vi "ReversedEngineering GetCaseStringConstants.vi"(0 "Diagram":refnum<vi>, 5 "error in (no error)":errorcluster) -> (15 "StringConstants":string[](array[string]), 16 "EventStructureUsed":bool, 19 "error out":errorcluster)   [LabVIEW 2012]
uses:
  <resource>/Framework/Providers/Open_GDS/UML/ReversedEngineering/ReversedEngineering QueuedStateMachinMemoryAction.ctl
panel:
  in  "Debug?":bool
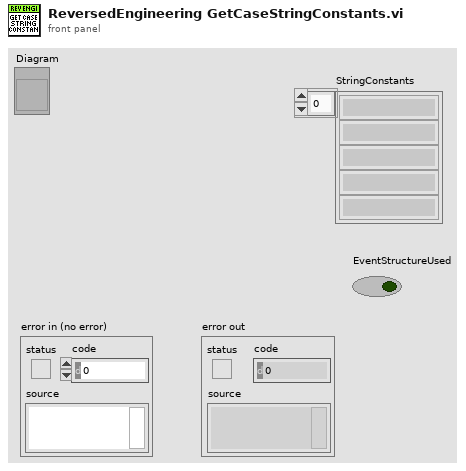
[diagram p1: front panel]
types:
  T1 = typedef "ReversedEngineering QueuedStateMachinMemoryAction.ctl" = enum16{"Initialize", "GetInsertQueuedArrayElementsVI", "SetQueuedStateJumps", "GetQueuedStateJumps"}
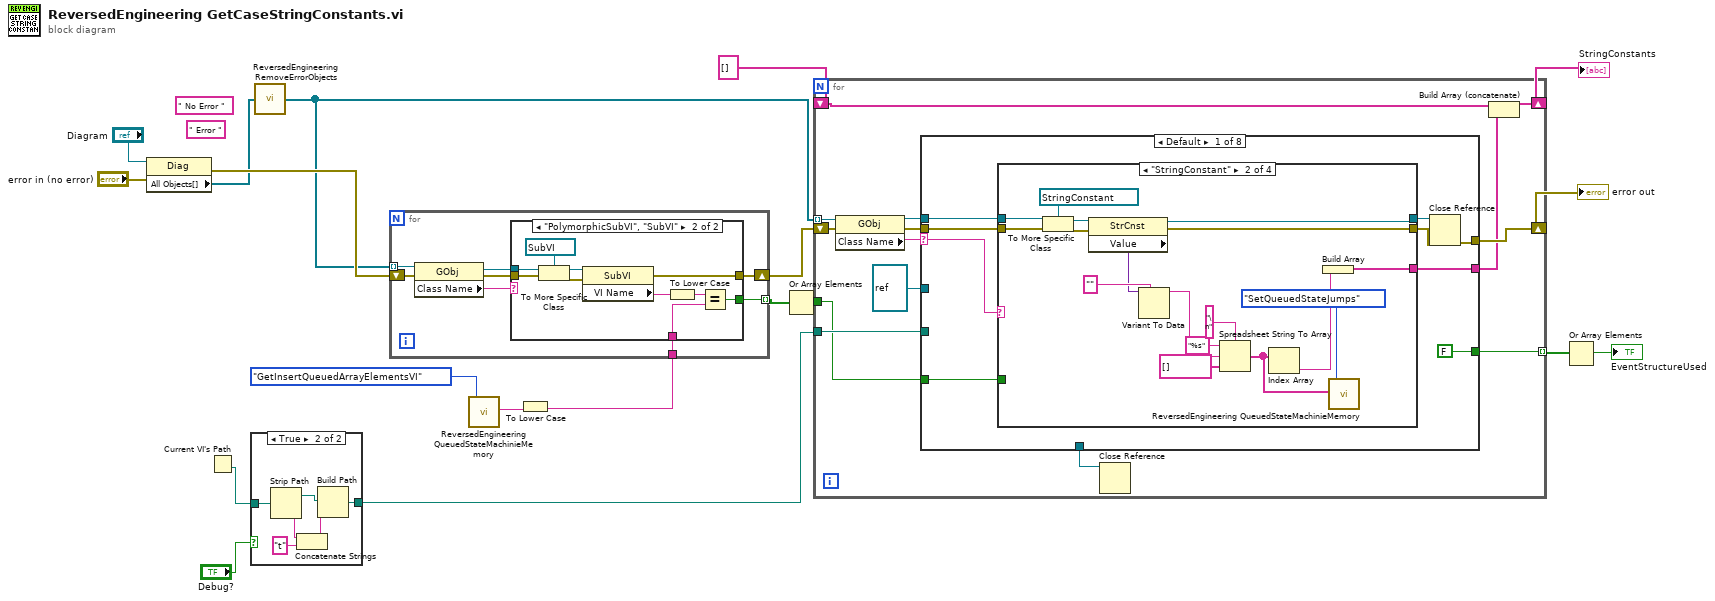
[diagram p0: block diagram]
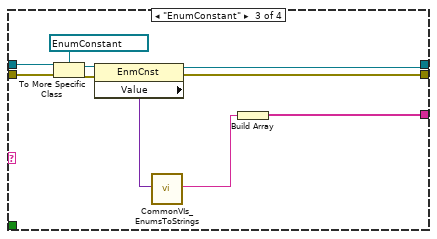
[diagram p5: hidden frame]
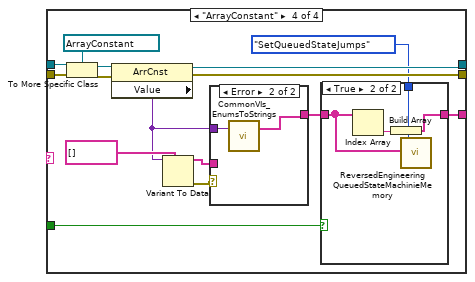
[diagram p6: hidden frame]
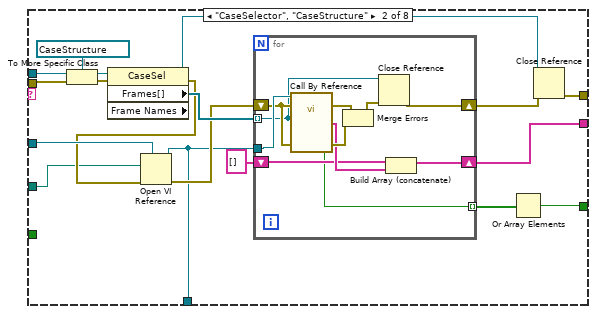
[diagram p9: hidden frame]
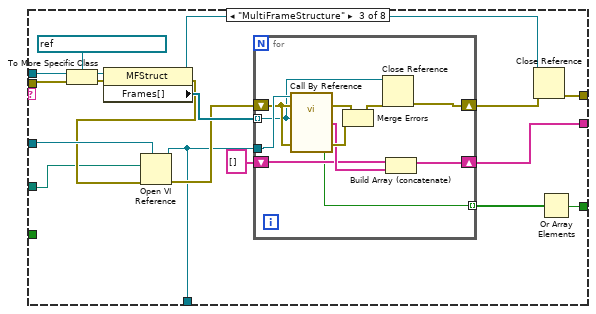
[diagram p10: hidden frame]
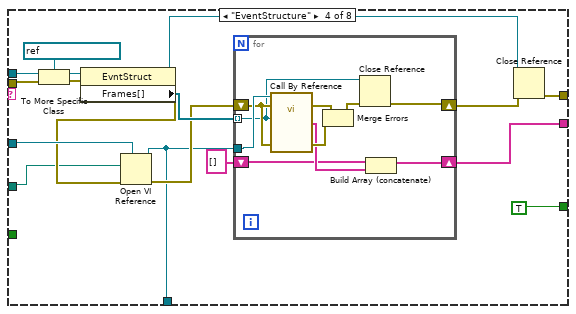
[diagram p11: hidden frame]
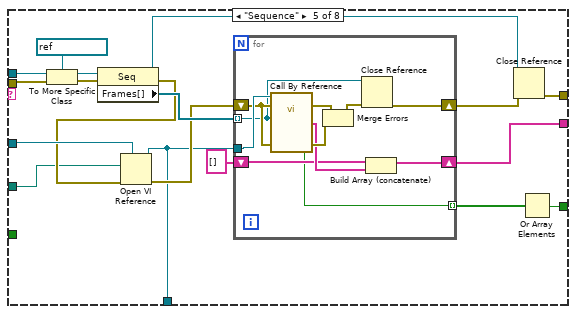
[diagram p12: hidden frame]
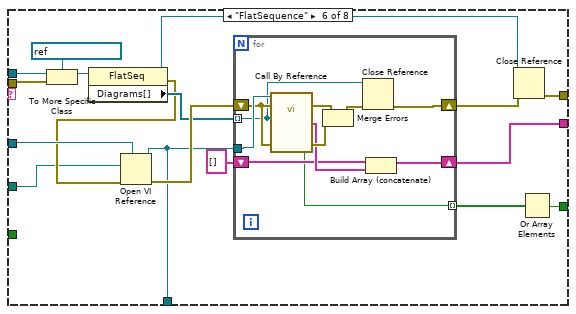
[diagram p13: hidden frame]
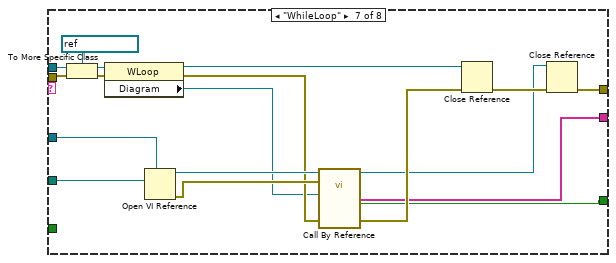
[diagram p14: hidden frame]
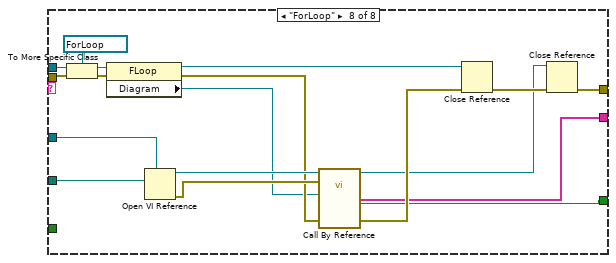
[diagram p15: hidden frame]
diagram:
  (unwired) " Error "
  (unwired) " No Error "
  n1 = property class="Diag"(reference="Diagram", error in="error in (no error)") -> (error out=w6:errorcluster, "All Objects[]"=w2:refnum<vi>[])  [unwired: 1 out]
  n2 = Current VI's Path() -> (path=w14:path)
  n3 = case shown="True" "Debug?" {
    tunnel: w14 -> [w20 w25]
    tunnel: [w20 w24] -> w13
    frame False {
    }
    frame True {
      n4 = Strip Path(path=w25) -> (stripped path=w26:path, name=w23:string)
      n5 = Concatenate Strings(w23, "t" ("string")) -> (w22:string)
      n6 = Build Path(base path=w26, name or relative path=w22) -> (appended path=w24:path)
    }
  }
  n7 = call <resource>:"ReversedEngineering RemoveErrorObjects.vi"("ObjectsIn"=w2) -> ("ObjectsOut"=w1:refnum<vi>[])
  n8 = call <resource>:"ReversedEngineering QueuedStateMachinieMemory.vi"("Action(GetInsertQueuedArrayElementsVI)"=ReversedEngineering_QueuedStateMachinMemoryAction."GetInsertQueuedArrayElementsVI" ("Action(GetInsertQueuedArrayElements)")) -> ("VIName"=w8:string)  [unwired: 3 in, 15 out]
  n9 = To Lower Case(string=w8) -> (all lower case string=w7:string)
  n10 = for {
    tunnel: w1 -> [w34] mode=indexing
    shift-right: [w27] -> w5
    shift-left: w6 -> [w32]
    tunnel: w7 -> [w29]
    tunnel: [w28] -> w4 mode=indexing
    n11 = property class="GObj"(reference=w34, error in=w32) -> (reference out=w31:refnum<vi>, error out=w30:errorcluster, "Class Name"=w33:string)
    n12 = case shown="\"PolymorphicSubVI\", \"SubVI\"" w33 {
      tunnel: w31 -> [_ w45]
      tunnel: w30 -> [w35 w43]
      tunnel: w29 -> [_ w39]
      tunnel: [_ w38] -> w28
      tunnel: [w35 w37] -> w27
      frame "False", Default {
      }
      frame "PolymorphicSubVI", "SubVI" {
        n13 = To More Specific Class(target class=refnum<vi> refnum ("WhileLoop"), reference=w45, error in=w43) -> (specific class reference=w42:refnum<vi>, error out=w36:errorcluster)
        n14 = property class="SubVI"(reference=w42, error in=w36) -> (error out=w37:errorcluster, "VI Name"=w41:string)  [unwired: 1 out]
        n15 = To Lower Case(string=w41) -> (all lower case string=w40:string)
        n16 = Equal?(x=w40, y=w39) -> (x = y?=w38:bool)
      }
    }
  }
  n17 = Or Array Elements(Boolean array=w4) -> (logical OR=w3:bool)
  n18 = for {
    tunnel: w1 -> [w59] mode=indexing
    shift-right: [w54] -> w17
    shift-left: w5 -> [w56]
    shift-right: [w52] -> w16
    shift-left: string[] [] -> [w53]
    tunnel: w13 -> [w49]
    tunnel: [w47] -> w11 mode=indexing
    tunnel: w3 -> [w46]
    n19 = property class="GObj"(reference=w59, error in=w56) -> (reference out=w57:refnum<vi>, error out=w55:errorcluster, "Class Name"=w58:string)
    n20 = case shown="Default" w58 {
      selector: w58 -> [w67 _ _ _ _ _ _ _]
      tunnel: w57 -> [w65 w138 w167 w195 w223 w251 w280 w298]
      tunnel: w55 -> [w66 w133 w163 w192 w219 w250 w274 w292]
      tunnel: [w68 w132 w162 w191 w218 w249 w266 w284] -> w54
      tunnel: [w62 w126 w156 w185 w213 w245 w269 w287] -> w51
      tunnel: refnum<vi> refnum ("VI Refnum") -> [_ w129 w159 w188 w215 w247 w268 w286]
      tunnel: w49 -> [_ w124 w153 w182 w210 w238 w264 w282]
      tunnel: [_ w123 w152 w181 w208 w237 _ _] -> w48
      tunnel: [FALSE ("EventStructureUsed") w121 w151 TRUE w207 w236 w263 w281] -> w47
      tunnel: w46 -> [w60 _ _ _ _ _ _ _]
      frame Default {
        n21 = case shown="\"StringConstant\"" w67 {
          tunnel: w66 -> [w70 w85 w95 w110]
          tunnel: w65 -> [w69 w86 w96 w111]
          tunnel: [w70 w82 w92 w108] -> w64
          tunnel: [w69 w81 w91 w107] -> w63
          tunnel: [_ w83 w93 w99] -> w62
          tunnel: w60 -> [_ _ _ w101]
          frame "False", Default {
          }
          frame "StringConstant" {
            n22 = To More Specific Class(target class=refnum<vi> refnum ("WhileLoop"), reference=w86, error in=w85) -> (specific class reference=w84:refnum<vi>, error out=w80:errorcluster)
            n23 = property class="StrCnst"(reference=w84, error in=w80) -> (reference out=w81:refnum<vi>, error out=w82:errorcluster, "Value"=w78:variant)
            n24 = Variant To Data(type="", Variant=w78) -> (data=w74:string)  [unwired: 1 in, 1 out]
            n25 = Spreadsheet String To Array(delimiter (Tab)="\n", format string="%s", spreadsheet string=w74, array type (2D Dbl)=string[] []) -> (array=w72:string[])
            n26 = Index Array(array=w72) -> (element=w73:string)  [unwired: 1 in]
            n27 = Build Array(w73) -> (w83:string[])
            n28 = call <resource>:"ReversedEngineering QueuedStateMachinieMemory.vi"("StateJumps"=w72, "Action(GetInsertQueuedArrayElementsVI)"=ReversedEngineering_QueuedStateMachinMemoryAction."SetQueuedStateJumps") -> ()  [unwired: 2 in, 16 out]
          }
          frame "EnumConstant" {
            n29 = To More Specific Class(target class=refnum<vi> refnum ("WhileLoop"), reference=w96, error in=w95) -> (specific class reference=w94:refnum<vi>, error out=w90:errorcluster)
            n30 = property class="EnmCnst"(reference=w94, error in=w90) -> (reference out=w91:refnum<vi>, error out=w92:errorcluster, "Value"=w89:variant)
            n31 = call <resource>:"CommonVIs_EnumsToStrings.vi"("SingleEnumVariantIn"=w89) -> ("EnumItem"=w88:string)  [unwired: 2 in, 16 out]
            n32 = Build Array(w88) -> (w93:string[])
          }
          frame "ArrayConstant" {
            n33 = To More Specific Class(target class=refnum<vi> refnum ("WhileLoop"), reference=w111, error in=w110) -> (specific class reference=w109:refnum<vi>, error out=w106:errorcluster)
            n34 = property class="ArrCnst"(reference=w109, error in=w106) -> (reference out=w107:refnum<vi>, error out=w108:errorcluster, "Value"=w103:variant)
            n35 = Variant To Data(type=string[] [], Variant=w103) -> (data=w102:string[], error out=w104:errorcluster)  [unwired: 1 in]
            n36 = case shown="Error" w104 {
              tunnel: w103 -> [_ w120]
              tunnel: w102 -> [w118 _]
              tunnel: [w118 w119] -> w100
              frame No Error {
              }
              frame Error {
                n37 = call <resource>:"CommonVIs_EnumsToStrings.vi"("ArrayEnumVariantIn"=w120) -> ("EnumItems(string)"=w119:string[])  [unwired: 2 in, 16 out]
              }
            }
            n38 = case shown="True" w101 {
              tunnel: w100 -> [w113 w115]
              tunnel: [w113 w116] -> w99
              tunnel: ReversedEngineering_QueuedStateMachinMemoryAction."SetQueuedStateJumps" ("Action(GetInsertQueuedArrayElementsVI)") -> [_ w117]
              frame False {
              }
              frame True {
                n39 = Index Array(array=w115) -> (element=w114:string)  [unwired: 1 in]
                n40 = Build Array(w114) -> (w116:string[])
                n41 = call <resource>:"ReversedEngineering QueuedStateMachinieMemory.vi"("StateJumps"=w115, "Action(GetInsertQueuedArrayElementsVI)"=w117) -> ()  [unwired: 2 in, 16 out]
              }
            }
          }
        }
        n42 = Close Reference(reference=w63, error in (no error)=w64) -> (error out=w68:errorcluster)
      }
      frame "CaseSelector", "CaseStructure" {
        n43 = To More Specific Class(target class=refnum<vi> refnum ("CaseSelector"), reference=w138, error in=w133) -> (specific class reference=w136:refnum<vi>, error out=w134:errorcluster)
        n44 = property class="CaseSel" props=["Frames[]", "Frame Names"](reference=w136, error in=w134) -> (reference out=w130:refnum<vi>, error out=w128:errorcluster, "Frames[]"=w135:refnum<vi>[])  [unwired: 1 out]
        n45 = Open VI Reference(type specifier VI Refnum (for type only)=w129, vi path=w124, error in (no error)=w128) -> (vi reference=w123:refnum<vi>, error out=w131:errorcluster)  [unwired: 3 out]
        n46 = for {
          tunnel: w135 -> [w140] mode=indexing
          shift-right: [w142] -> w127
          shift-left: w131 -> [w147]
          tunnel: w123 -> [w148]
          shift-right: [w143] -> w126
          shift-left: string[] [] -> [w144]
          tunnel: [w139] -> w122 mode=indexing
          n47 = call-by-ref "?"(reference=w148, error in=w147, "Diagram"=w140, "error in (no error)"=w147) -> (error out=w149:errorcluster, "StringConstants"=w145:string[], "EventStructureUsed"=w139:bool, 19:"error out"=w146:errorcluster)  [unwired: 15 in, 1 out]
          n48 = Merge Errors(w149, w146) -> (w141:errorcluster)
          n49 = Close Reference(reference=w140, error in (no error)=w141) -> (error out=w142:errorcluster)
          n50 = Build Array (concatenate)(w144, w145) -> (w143:string[])
        }
        n51 = Or Array Elements(Boolean array=w122) -> (logical OR=w121:bool)
        n52 = Close Reference(reference=w130, error in (no error)=w127) -> (error out=w132:errorcluster)
      }
      frame "MultiFrameStructure" {
        n53 = To More Specific Class(target class=refnum<vi> refnum ("MultiFrameStructure"), reference=w167, error in=w163) -> (specific class reference=w166:refnum<vi>, error out=w164:errorcluster)
        n54 = property class="MFStruct"(reference=w166, error in=w164) -> (reference out=w160:refnum<vi>, error out=w158:errorcluster, "Frames[]"=w165:refnum<vi>[])
        n55 = Open VI Reference(type specifier VI Refnum (for type only)=w159, vi path=w153, error in (no error)=w158) -> (vi reference=w152:refnum<vi>, error out=w161:errorcluster)  [unwired: 3 out]
        n56 = for {
          tunnel: w165 -> [w171] mode=indexing
          shift-right: [w169] -> w157
          shift-left: w161 -> [w176]
          tunnel: w152 -> [w177]
          shift-right: [w172] -> w156
          shift-left: string[] [] -> [w173]
          tunnel: [w168] -> w150 mode=indexing
          n57 = call-by-ref "?"(reference=w177, error in=w176, "Diagram"=w171, "error in (no error)"=w176) -> (error out=w178:errorcluster, "StringConstants"=w174:string[], "EventStructureUsed"=w168:bool, 19:"error out"=w175:errorcluster)  [unwired: 15 in, 1 out]
          n58 = Merge Errors(w178, w175) -> (w170:errorcluster)
          n59 = Close Reference(reference=w171, error in (no error)=w170) -> (error out=w169:errorcluster)
          n60 = Build Array (concatenate)(w173, w174) -> (w172:string[])
        }
        n61 = Close Reference(reference=w160, error in (no error)=w157) -> (error out=w162:errorcluster)
        n62 = Or Array Elements(Boolean array=w150) -> (logical OR=w151:bool)
      }
      frame "EventStructure" {
        n63 = To More Specific Class(target class=refnum<vi> refnum ("EventStructure"), reference=w195, error in=w192) -> (specific class reference=w180:refnum<vi>, error out=w193:errorcluster)
        n64 = property class="EvntStruct"(reference=w180, error in=w193) -> (reference out=w189:refnum<vi>, error out=w187:errorcluster, "Frames[]"=w194:refnum<vi>[])
        n65 = Open VI Reference(type specifier VI Refnum (for type only)=w188, vi path=w182, error in (no error)=w187) -> (vi reference=w181:refnum<vi>, error out=w190:errorcluster)  [unwired: 3 out]
        n66 = for {
          tunnel: w194 -> [w196] mode=indexing
          shift-right: [w197] -> w186
          shift-left: w190 -> [w203]
          tunnel: w181 -> [w204]
          shift-right: [w199] -> w185
          shift-left: string[] [] -> [w200]
          n67 = call-by-ref "?"(reference=w204, error in=w203, "Diagram"=w196, "error in (no error)"=w203) -> (error out=w205:errorcluster, "StringConstants"=w201:string[], 19:"error out"=w202:errorcluster)  [unwired: 15 in, 2 out]
          n68 = Merge Errors(w205, w202) -> (w198:errorcluster)
          n69 = Close Reference(reference=w196, error in (no error)=w198) -> (error out=w197:errorcluster)
          n70 = Build Array (concatenate)(w200, w201) -> (w199:string[])
        }
        n71 = Close Reference(reference=w189, error in (no error)=w186) -> (error out=w191:errorcluster)
      }
      frame "Sequence" {
        n72 = To More Specific Class(target class=refnum<vi> refnum ("Sequence"), reference=w223, error in=w219) -> (specific class reference=w222:refnum<vi>, error out=w220:errorcluster)
        n73 = property class="Seq"(reference=w222, error in=w220) -> (reference out=w216:refnum<vi>, error out=w214:errorcluster, "Frames[]"=w221:refnum<vi>[])
        n74 = Open VI Reference(type specifier VI Refnum (for type only)=w215, vi path=w210, error in (no error)=w214) -> (vi reference=w208:refnum<vi>, error out=w217:errorcluster)  [unwired: 3 out]
        n75 = for {
          tunnel: w221 -> [w225] mode=indexing
          shift-right: [w227] -> w209
          shift-left: w217 -> [w232]
          tunnel: w208 -> [w233]
          shift-right: [w228] -> w213
          shift-left: string[] [] -> [w229]
          tunnel: [w224] -> w206 mode=indexing
          n76 = call-by-ref "?"(reference=w233, error in=w232, "Diagram"=w225, "error in (no error)"=w232) -> (error out=w234:errorcluster, "StringConstants"=w230:string[], "EventStructureUsed"=w224:bool, 19:"error out"=w231:errorcluster)  [unwired: 15 in, 1 out]
          n77 = Merge Errors(w234, w231) -> (w226:errorcluster)
          n78 = Close Reference(reference=w225, error in (no error)=w226) -> (error out=w227:errorcluster)
          n79 = Build Array (concatenate)(w229, w230) -> (w228:string[])
        }
        n80 = Close Reference(reference=w216, error in (no error)=w209) -> (error out=w218:errorcluster)
        n81 = Or Array Elements(Boolean array=w206) -> (logical OR=w207:bool)
      }
      frame "FlatSequence" {
        n82 = To More Specific Class(target class=refnum<vi> refnum ("FlatSequence"), reference=w251, error in=w250) -> (specific class reference=w242:refnum<vi>)  [unwired: 1 out]
        n83 = property class="FlatSeq"(reference=w242) -> (reference out=w239:refnum<vi>, error out=w240:errorcluster, "Diagrams[]"=w241:refnum<vi>[])  [unwired: 1 in]
        n84 = Open VI Reference(type specifier VI Refnum (for type only)=w247, vi path=w238, error in (no error)=w240) -> (vi reference=w237:refnum<vi>, error out=w248:errorcluster)  [unwired: 3 out]
        n85 = for {
          tunnel: w241 -> [w253] mode=indexing
          shift-right: [w255] -> w246
          shift-left: w248 -> [w260]
          tunnel: w237 -> [w261]
          shift-right: [w256] -> w245
          shift-left: string[] [] -> [w257]
          tunnel: [w252] -> w235 mode=indexing
          n86 = call-by-ref "?"(reference=w261, error in=w260, "Diagram"=w253, "error in (no error)"=w260) -> (error out=w262:errorcluster, "StringConstants"=w258:string[], "EventStructureUsed"=w252:bool, 19:"error out"=w259:errorcluster)  [unwired: 15 in, 1 out]
          n87 = Merge Errors(w262, w259) -> (w254:errorcluster)
          n88 = Close Reference(reference=w253, error in (no error)=w254) -> (error out=w255:errorcluster)
          n89 = Build Array (concatenate)(w257, w258) -> (w256:string[])
        }
        n90 = Close Reference(reference=w239, error in (no error)=w246) -> (error out=w249:errorcluster)
        n91 = Or Array Elements(Boolean array=w235) -> (logical OR=w236:bool)
      }
      frame "WhileLoop" {
        n92 = To More Specific Class(target class=refnum<vi> refnum ("WhileLoop"), reference=w280, error in=w274) -> (specific class reference=w279:refnum<vi>, error out=w275:errorcluster)
        n93 = property class="WLoop"(reference=w279, error in=w275) -> (reference out=w277:refnum<vi>, error out=w271:errorcluster, "Diagram"=w270:refnum<vi>)
        n94 = Open VI Reference(type specifier VI Refnum (for type only)=w268, vi path=w264) -> (vi reference=w273:refnum<vi>, error out=w276:errorcluster)  [unwired: 1 in, 3 out]
        n95 = call-by-ref "?"(reference=w273, error in=w276, "Diagram"=w270, "error in (no error)"=w271) -> (reference out=w265:refnum<vi>, "StringConstants"=w269:string[], "EventStructureUsed"=w263:bool, "error out"=w272:errorcluster)  [unwired: 15 in, 1 out]
        n96 = Close Reference(reference=w277, error in (no error)=w272) -> (error out=w267:errorcluster)
        n97 = Close Reference(reference=w265, error in (no error)=w267) -> (error out=w266:errorcluster)
      }
      frame "ForLoop" {
        n98 = To More Specific Class(target class=refnum<vi> refnum ("WhileLoop"), reference=w298, error in=w292) -> (specific class reference=w297:refnum<vi>, error out=w293:errorcluster)
        n99 = property class="FLoop"(reference=w297, error in=w293) -> (reference out=w295:refnum<vi>, error out=w289:errorcluster, "Diagram"=w288:refnum<vi>)
        n100 = Open VI Reference(type specifier VI Refnum (for type only)=w286, vi path=w282) -> (vi reference=w291:refnum<vi>, error out=w294:errorcluster)  [unwired: 1 in, 3 out]
        n101 = call-by-ref "?"(reference=w291, error in=w294, "Diagram"=w288, "error in (no error)"=w289) -> (reference out=w283:refnum<vi>, "StringConstants"=w287:string[], "EventStructureUsed"=w281:bool, "error out"=w290:errorcluster)  [unwired: 15 in, 1 out]
        n102 = Close Reference(reference=w295, error in (no error)=w290) -> (error out=w285:errorcluster)
        n103 = Close Reference(reference=w283, error in (no error)=w285) -> (error out=w284:errorcluster)
      }
    }
    n104 = Close Reference(reference=w48) -> ()  [unwired: 1 in, 1 out]
    n105 = Build Array (concatenate)(w53, w51) -> (w52:string[])
  }
  "error out" <- w17
  "StringConstants" <- w16
  n106 = Or Array Elements(Boolean array=w11) -> (logical OR=→"EventStructureUsed":bool)
